vi "Square Inputs.vi"(9 "Before Square":dbl, 10 "Square Inputs":bool) -> (1 "After Square":dbl)   [LabVIEW 2014, in "Joystick.lvlib"]
uses:
  Joystick.lvlib
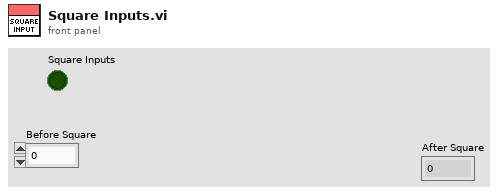
[diagram p1: front panel]
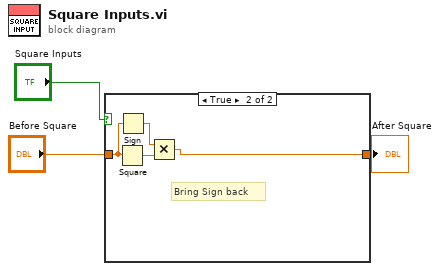
[diagram p0: block diagram]
diagram:
  n1 = case shown="True" "Square Inputs" {
    tunnel: "Before Square" -> [w4 w7]
    tunnel: [w4 w6] -> w1
    frame False {
    }
    frame True {
      # "Bring Sign back"
      n2 = Square(x=w7) -> (x^2=w8:dbl)
      n3 = Sign(1:w7) -> (0:w5:dbl)
      n4 = Multiply(x=w5, y=w8) -> (x*y=w6:dbl)
    }
  }
  "After Square" <- w1
